vi "ESP Read.vi"(4 "error in":errorcluster, 7 "Address / Port":i16=1 min=1 max=31 step=1) -> (0 "error out":errorcluster, 1 "Response String":string, 3 "Address / Port dup":i16=1 min=1 max=31 step=1)   [LabVIEW 2014]
panel:
  out "status":bool[](array[boolean])
  out "byte count":i32
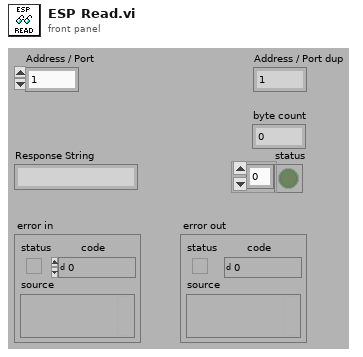
[diagram p1: front panel]
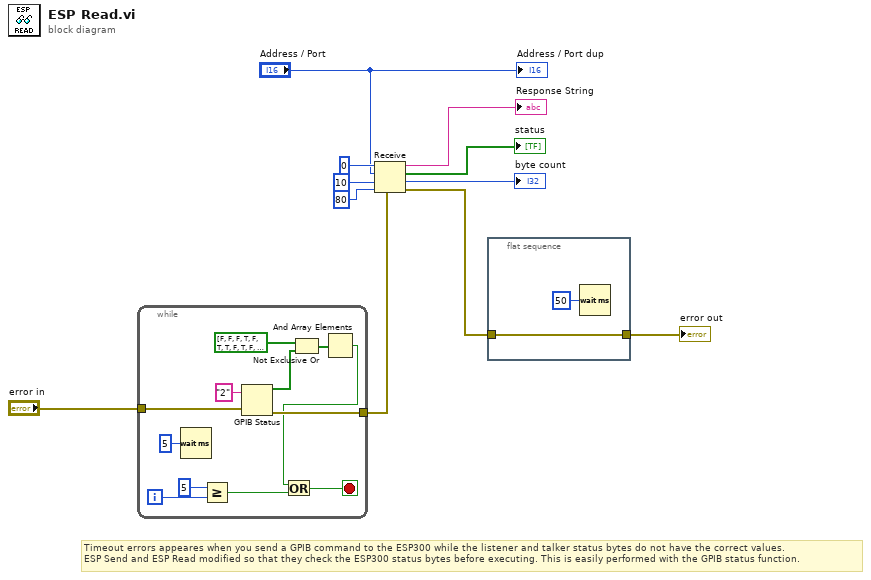
[diagram p0: block diagram]
diagram:
  # "Timeout errors appeares when you send a GPIB command to the ESP300 while the listener and talker status bytes do not have the correct values.\nESP Send and ESP Read modified so that they check the ESP300 status bytes before executing. This is easily performed with the GPIB status function."
  n1 = while {
    tunnel: "error in" -> [w22]
    tunnel: [w21] -> w3
    i -> [w20]
    stop <- w17 stop-if-true
    n2 = Wait (ms)(milliseconds to wait=u32 5) -> ()  [unwired: 1 out]
    n3 = Greater Or Equal?(x=5, y=w20) -> (x >= y?=w18:bool)
    n4 = GPIB Status(0:"2" ("address string"), 1:w22) -> (2:w15:bool[], 5:w21:errorcluster)  [unwired: 2 out]
    n5 = Not Exclusive Or(1:w15, 2:bool[] [FALSE, FALSE, FALSE, TRUE, FALSE, TRUE, TRUE, FALSE, TRUE, FALSE, FALSE, FALSE, FALSE, FALSE, FALSE, FALSE] ("status 2")) -> (0:w14:bool[])
    n6 = And Array Elements(Boolean array=w14) -> (logical AND=w13:bool)
    n7 = Or(x=w13, y=w18) -> (x .or. y?=w17:bool)
  }
  n8 = Receive(4:w3, 6:80 ("count"), 7:i16 10 ("mode"), 8:"Address / Port", 9:0 ("bus")) -> (0:w2:errorcluster, 1:→"byte count":i32, 2:→"status":bool[], 3:→"Response String":string)
  n9 = flat-sequence {
    tunnel: w2 -> [w24]
    tunnel: [w24] -> w1
    frame #0 {
      n10 = Wait (ms)(milliseconds to wait=u32 50) -> ()  [unwired: 1 out]
    }
  }
  "error out" <- w1
  "Address / Port dup" <- "Address / Port"
